vi "Install 1.0.vi"   [LabVIEW 2020, in "nisyscfg.lvlib"]
doc: "Performs an install or uninstall of software on an RT system."
uses:
  <vilib>/nisyscfg/nisyscfg.lvlib
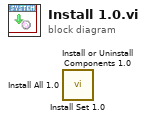
[diagram p0: block diagram]
diagram:
  n1 = call <vilib>:"Install Set 1.0.vi"() -> ()  [unwired: 9 in, 3 out]
  n2 = call <vilib>:"Install or Uninstall Components 1.0.vi"() -> ()  [unwired: 9 in, 3 out]
  n3 = call <vilib>:"Install All 1.0.vi"() -> ()  [unwired: 8 in, 4 out]
